vi "set_z-intensity_tuples.vi"(8 "error in (no error)":errorcluster, 10 "z/intensity tuples (1st row: z values, 2nd row intensity values)":i16[][](array[numeric]), 11 "FPGAWrapperAK101022Resonance in":refnum<class "FPGAWrapperAK101022Resonance.lvclass">) -> (0 "error out":errorcluster, 3 "FPGAWrapperAK101022Resonance out":refnum<class "FPGAWrapperAK101022Resonance.lvclass">)   [LabVIEW 2010, in "FPGAWrapperAK101022Resonance.lvclass"]
uses:
  FPGAWrapperAK101022Resonance.lvclass
  scan_specification_cluster.ctl
  class_data.vi
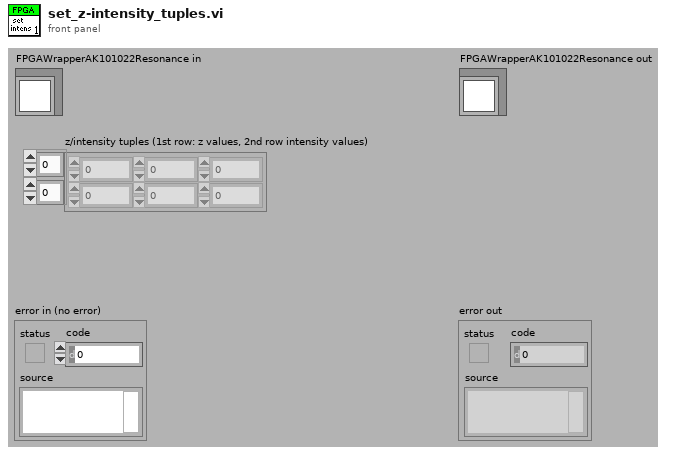
[diagram p1: front panel]
types:
  T1 = typedef "scan_specification_cluster.ctl" = cluster{"x amplitude":u16, "x resolution (pixels)":u16, "x offset fly-forward (iterations)":u16, "x offset fly-back (iterations)":u16, "y resolution (nr. of lines)":u16, "y step size":u16, "iterations per pixel":u16, "number of frames":i32, "y offset (pixels)":u16, "number of y-brake lines  (before y-fly-back)":u16, "number y-brake lines (after y-fly-back)":u16, "number of y-fly-back steps":u16, "lines per z step":u16, "number of z/intensity tuples":u16}
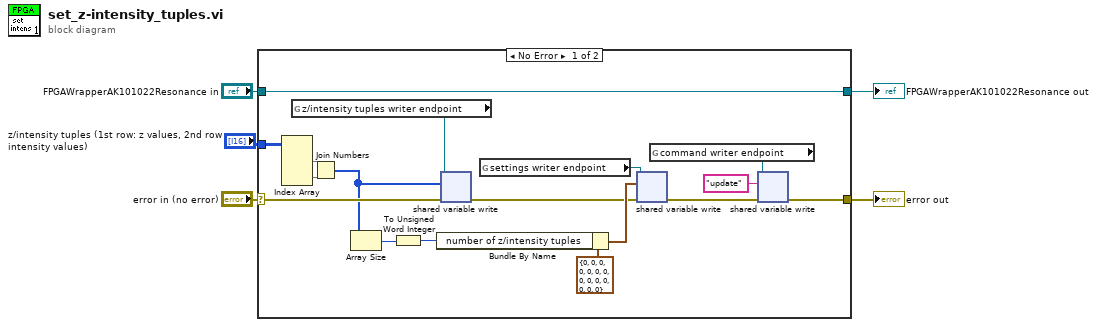
[diagram p0: block diagram]
diagram:
  n1 = case shown="No Error" "error in (no error)" {
    selector: "error in (no error)" -> [w12 w24]
    tunnel: [w19 w24] -> w4
    tunnel: [w22 w23] -> w2
    tunnel: "FPGAWrapperAK101022Resonance in" -> [w22 w23]
    tunnel: "z/intensity tuples (1st row: z values, 2nd row intensity values)" -> [w6 _]
    frame No Error {
      n2 = Index Array(array=w6) -> (element #1=w9:i16[], element #2=w8:i16[])  [unwired: 4 in]
      n3 = global read "class_data.vi" "z/intensity tuples writer endpoint"() -> (w10:refnum<k21>)
      n4 = Join Numbers(hi=w9, lo=w8) -> ((hi.lo)=w7:u32[])
      n5 = Array Size(array=w7) -> (size(s)=w15:i32)
      n6 = To Unsigned Word Integer(number=w15) -> (unsigned 16bit integer=w14:u16)
      n7 = Bundle By Name(cluster=T1 {"x amplitude"=0, "x resolution (pixels)"=0, "x offset fly-forward (iterations)"=0, "x offset fly-back (iterations)"=0, "y resolution (nr. of lines)"=0, "y step size"=0, "iterations per pixel"=0, "number of frames"=0, "y offset (pixels)"=0, "number of y-brake lines  (before y-fly-back)"=0, "number y-brake lines (after y-fly-back)"=0, "number of y-fly-back steps"=0, "lines per z step"=0, "number of z/intensity tuples"=0} ("scan specification"), "number of z/intensity tuples"=w14) -> (w17:T1)
      n8 = shared-variable-write(w10, w12, w7) -> (w11:errorcluster)  [unwired: 1 in, 2 out]
      n9 = global read "class_data.vi" "settings writer endpoint"() -> (w18:refnum<k21>)
      n10 = shared-variable-write(w18, w11, w17) -> (w13:errorcluster)  [unwired: 1 in, 2 out]
      n11 = global read "class_data.vi" "command writer endpoint"() -> (w21:refnum<k21>)
      n12 = shared-variable-write(w21, w13, "update" ("data in")) -> (w19:errorcluster)  [unwired: 1 in, 2 out]
    }
    frame Error {
    }
  }
  "error out" <- w4
  "FPGAWrapperAK101022Resonance out" <- w2
